vi "Aeroflex ATT Release.vi"(7 "Aeroflex ATT":T1, 8 "error in (no error)":errorcluster, 11 "DAQmx Dev Name (PAModule)":string) -> (0 "error out":errorcluster {"code" format="%.0x"})   [LabVIEW 2011]
uses:
  TypeDefs/Aeroflex ATT Instrument Info.ctl
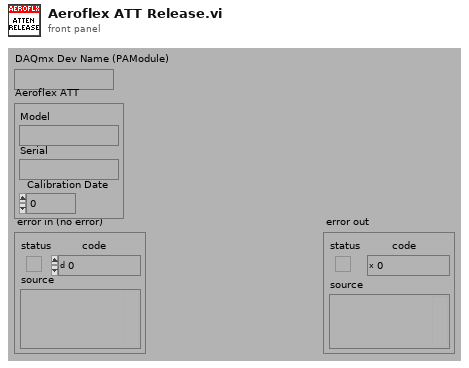
[diagram p1: front panel]
types:
  T1 = typedef "Aeroflex ATT Instrument Info.ctl" = cluster{"Model":string, "Serial":string, "Calibration Date":dbl}
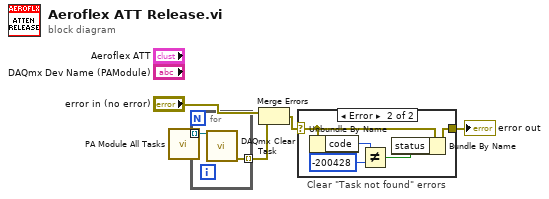
[diagram p0: block diagram]
diagram:
  n1 = call "PA Module All Tasks.vi"() -> ("Task Names"=w5:refnum<k21>[])  [unwired: 4 out]
  n2 = for {
    tunnel: [w7] -> w3 mode=indexing
    tunnel: w5 -> [w6] mode=indexing
    n3 = call <vilib>:"DAQmx Clear Task.vi"("task in"=w6) -> ("error out"=w7:errorcluster)  [unwired: 1 in, 13 out]
  }
  n4 = Merge Errors("error in (no error)", w3) -> (w2:errorcluster)
  n5 = case "Clear \"Task not found\" errors" shown="Error" w2 {
    selector: w2 -> [w8 w11]
    tunnel: [w8 w9] -> w1
    frame No Error {
    }
    frame Error {
      n6 = Unbundle By Name(w11) -> ("code"=w13:i32)
      n7 = Not Equal?(x=w13, y=-200428) -> (x != y?=w10:bool)
      n8 = Bundle By Name(cluster=w11, "status"=w10) -> (w9:errorcluster)
    }
  }
  "error out" <- w1
